vi "ISEG_HVBoard.set Refresh Status.vi"(0 "i ref in":refnum<vi>, 2 "Refresh Status":i32, 3 "Force":bool, 5 "error in (no error)":errorcluster) -> (14 "i ref out":refnum<vi>, 19 "error out":errorcluster)   [LabVIEW 2014, in "ISEG_HVBoard.lvlib"]
doc: "this vi set the default values for force_status and refresh rate."
uses:
  ISEG_HVBoard.lvlib
  CS_Core/CSSystem/CoreLib/CoreLib.string 2 byte array.vi
  CS_Core/CSSystem/CoreLib/CoreLib.short 2 byte array.vi
  CS_Core/CSSystem/CoreLib/CoreLib.double 2 byte array.vi
  CS_Core/CSSystem/CoreLib/CoreLib.lvlib
  CS_Core/BaseProcess/BaseProcess.lvlib
  CSlibraries-extern/DimLVEvent/LVDimInterface/LVDimInterface.lvlib
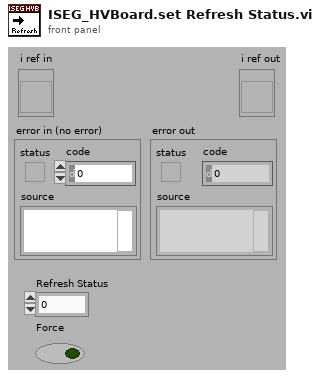
[diagram p1: front panel]
types:
  T1 = typedef "BaseProcess.lvlib/BaseProcess.i attribute.ctl" = cluster{"EventStatus":string, "EventError":i32, "PresetEvtWatchD":i32, "PresetPdcWatchD":i32, "EventTimeout":i32, "PeriodicInterval":i32, "Interface":string[], "Address":string[], "Special":string[], "PeriodicError":i32, "PeriodicStatus":string, "SuperProc":string, "Descriptors":T2[], "CaseRef":refnum<vi>, "PdcRef":refnum<vi>, "Thread Ref":refnum<vi>, "eventErrorID":i32, "eventStatusID":i32, "periodicErrorID":i32, "periodicStatusID":i32, "pdcCtrID":i32}
  T2 = typedef "BaseProcess.lvlib/BaseProcess.descriptor definition.ctl" = cluster{"selector":string, "descriptor":T3}
  T3 = typedef "BaseProcess.lvlib/BaseProcess.descriptor string definition.ctl" = string
  T4 = typedef "CoreDefs.rawDataType.ctl" = i8[]
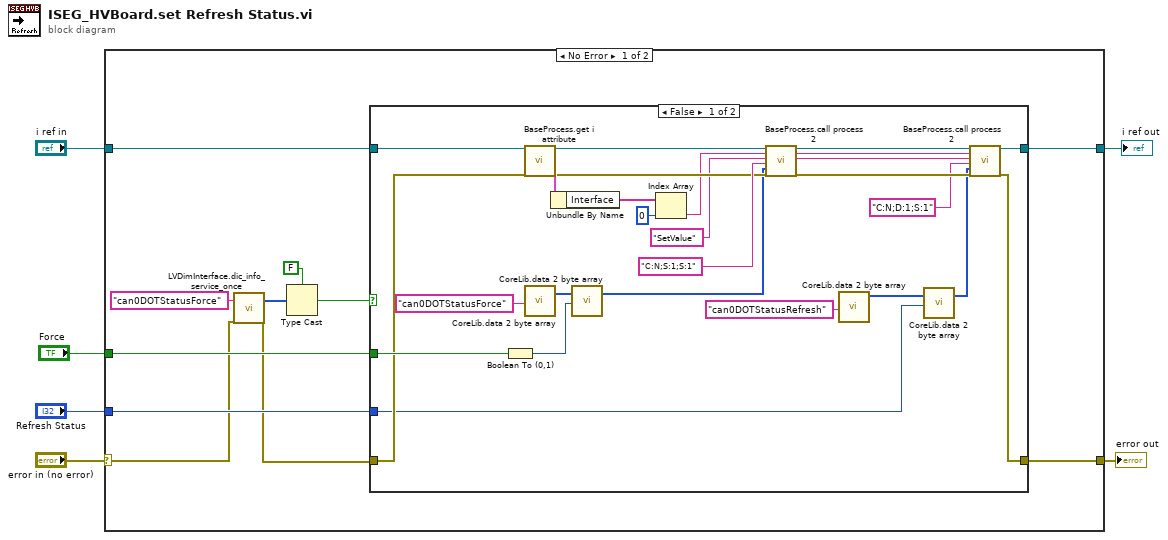
[diagram p0: block diagram]
diagram:
  n1 = case shown="No Error" "error in (no error)" {
    selector: "error in (no error)" -> [w8 w44]
    tunnel: "i ref in" -> [w17 w45]
    tunnel: "Refresh Status" -> [w16 _]
    tunnel: "Force" -> [w13 _]
    tunnel: [w15 w45] -> w2
    tunnel: [w14 w44] -> w1
    frame No Error {
      n2 = call "LVDimInterface.dic_info_service_once.vi"("serviceName"="can0DOTStatusForce", "error in (no error)"=w8) -> ("data"=w9:i8[], "error out"=w7:errorcluster)  [unwired: 14 in, 2 out]
      n3 = Type Cast(type=FALSE, x=w9) -> (*(type *) &x=w10:bool)
      n4 = case shown="False" w10 {
        tunnel: w17 -> [w41 w43]
        tunnel: w16 -> [w19 _]
        tunnel: [w33 w43] -> w15
        tunnel: [w31 w42] -> w14
        tunnel: w13 -> [w25 _]
        tunnel: w7 -> [w24 w42]
        frame False {
          w29 = "SetValue" ("Selector")
          n5 = Boolean To (0,1)(Boolean=w25) -> (0, 1=w23:i16)
          n6 = call "BaseProcess.get i attribute.vi"("i ref in"=w41, "error in (no error)"=w24) -> ("i ref out"=w36:refnum<vi>, "i attribute"=w38:T1, "error out"=w35:errorcluster)  [unwired: 15 in]
          n7 = call-poly "CoreLib.data 2 byte array.vi"("string"="can0DOTStatusForce") -> ("byteArray out"=w22:T4)  [unwired: 18 in]
          n8 = Unbundle By Name(w38) -> ("Interface"=w40:string[])
          n9 = call-poly "CoreLib.data 2 byte array.vi"("byteArray"=w22, "i16"=w23) -> ("byteArray out"=w21:T4)  [unwired: 17 in]
          n10 = Index Array(array=w40, index=0) -> (element=w30:string)
          n11 = call "BaseProcess.call process 2.vi"("i ref in"=w36, "Object"=w30, "Selector"=w29, "Data Descriptor"="C:N;S:1;S:1", "Data"=w21, "error in (no error)"=w35) -> ("i ref out"=w34:refnum<vi>, "error out"=w32:errorcluster)  [unwired: 12 in]
          n12 = call-poly "CoreLib.data 2 byte array.vi"("string"="can0DOTStatusRefresh") -> ("byteArray out"=w20:T4)  [unwired: 18 in]
          n13 = call-poly "CoreLib.data 2 byte array.vi"("byteArray"=w20, "f64"=w19) -> ("byteArray out"=w18:T4)  [unwired: 17 in]
          n14 = call "BaseProcess.call process 2.vi"("i ref in"=w34, "Object"=w30, "Selector"=w29, "Data Descriptor"="C:N;D:1;S:1", "Data"=w18, "error in (no error)"=w32) -> ("i ref out"=w33:refnum<vi>, "error out"=w31:errorcluster)  [unwired: 12 in]
        }
        frame True {
        }
      }
    }
    frame Error {
    }
  }
  "error out" <- w1
  "i ref out" <- w2
